vi "Open.vi"(8 "error in (no error)":errorcluster, 11 "MelsecTCP in":refnum<class "ModbusRtu.lvclass">) -> (0 "error out":errorcluster, 3 "MelsecTCP out":refnum<class "ModbusRtu.lvclass">)   [LabVIEW 2020, in "HslCommunication.lvlib" / "ModbusRtu.lvclass"]
uses:
  ModbusRtu.lvclass
  ModbusRtu.lvclass/ModbusRtu.ctl
  E:/Git/Libraries/develop/HslCommunication/_Dependenciecs/HslCommunication.dll
  _Dependenciecs/HslCommunication.dll
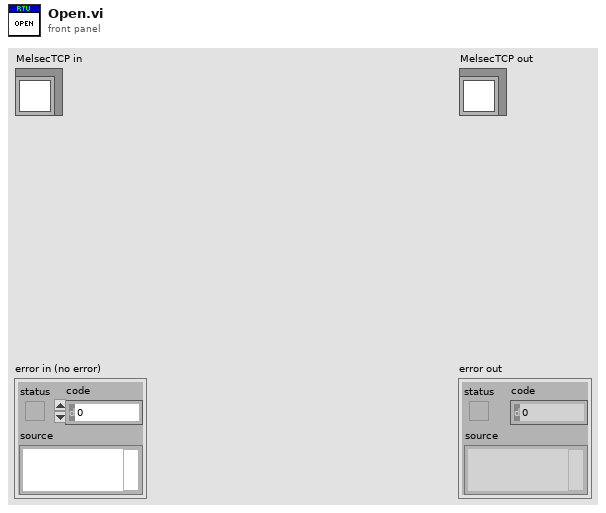
[diagram p1: front panel]
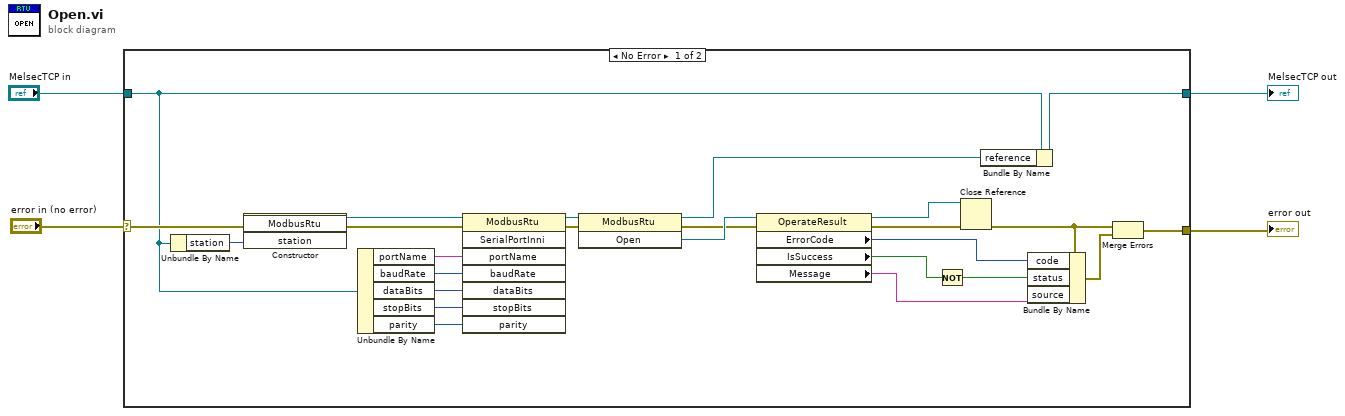
[diagram p0: block diagram]
diagram:
  n1 = case shown="No Error" "error in (no error)" {
    selector: "error in (no error)" -> [w18 w31]
    tunnel: "MelsecTCP in" -> [w7 w30]
    tunnel: [w29 w30] -> w1
    tunnel: [w24 w31] -> w2
    frame No Error {
      n2 = Unbundle By Name(w7) -> ("station"=w8:u8)
      n3 = constructor class="ModbusRtu"(error in=w18, "station"=w8) -> (reference out=w5:refnum<k24>, error out=w21:errorcluster)  [unwired: 2 in, 2 out]
      n4 = Unbundle By Name(w7) -> ("portName"=w9:string, "baudRate"=w13:i32, "dataBits"=w12:i32, "stopBits"=w11:i32, "parity"=w10:i32)
      n5 = invoke class="ModbusRtu" method="SerialPortInni"(reference=w5, error in=w21, "portName"=w9, "baudRate"=w13, "dataBits"=w12, "stopBits"=w11, "parity"=w10) -> (reference out=w19:refnum<k24>, error out=w16:errorcluster)  [unwired: 1 in, 6 out]
      n6 = invoke class="ModbusRtu" method="Open"(reference=w19, error in=w16) -> (reference out=w17:refnum<k24>, error out=w14:errorcluster, "Open"=w15:refnum<k24>)  [unwired: 1 in]
      n7 = property class="OperateResult"(reference=w15, error in=w14) -> (reference out=w23:refnum<k24>, error out=w22:errorcluster, "ErrorCode"=w27:i32, "IsSuccess"=w20:bool, "Message"=w25:string)
      n8 = Not(x=w20) -> (.not. x?=w26:bool)
      n9 = Close Reference(reference=w23, error in (no error)=w22) -> (error out=w6:errorcluster)
      n10 = Bundle By Name(cluster=w7, "reference"=w17) -> (w29:refnum<class "ModbusRtu.lvclass">)
      n11 = Bundle By Name(cluster=w6, "code"=w27, "status"=w26, "source"=w25) -> (w28:errorcluster)
      n12 = Merge Errors(w6, w28) -> (w24:errorcluster)
    }
    frame Error {
    }
  }
  "error out" <- w2
  "MelsecTCP out" <- w1
